vi "close excel file if open.vi"(8 "error in (no error)":errorcluster, 11 "report file path in":path) -> (0 "error out":errorcluster, 3 "report file path out":path)   [LabVIEW 2016]
uses:
  <vilib>/Utility/NIReport.llb/NI_report.lvclass
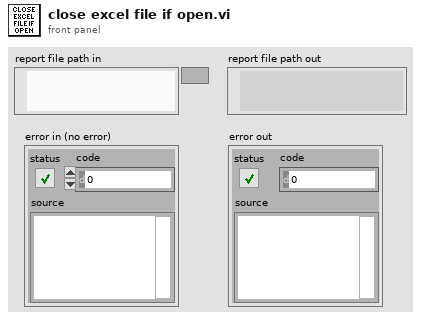
[diagram p1: front panel]
types:
  T1 = enum16{"maximized", "minimized", "normal", "no change"}
  T2 = enum16{"Standard Report", "HTML", "Word", "Excel"}
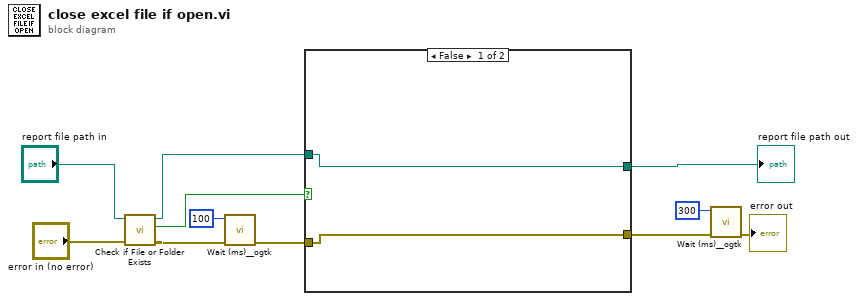
[diagram p0: block diagram]
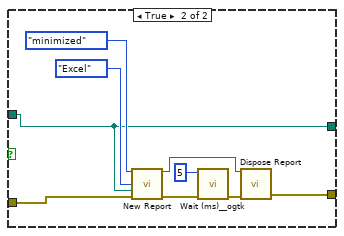
[diagram p2: hidden frame]
diagram:
  n1 = call <vilib>:"Check if File or Folder Exists.vi"("error in (no error)"="error in (no error)", "path"="report file path in") -> ("error out"=w5:errorcluster, "file or folder exists?"=w4:bool, "dup path"=w2:path)  [unwired: 7 in]
  n2 = call "Wait (ms)__ogtk.vi"("error in (no error)"=w5, "milliseconds to wait"=u32 100) -> ("error out"=w7:errorcluster)  [unwired: 8 in, 1 out]
  n3 = case shown="False" w4 {
    tunnel: [w12 w16] -> w11
    tunnel: w7 -> [w12 w15]
    tunnel: w2 -> [w13 w14]
    tunnel: [w13 w14] -> w1
    frame False {
    }
    frame True {
      n4 = call <vilib>:"New Report.vi"("window state (normal)"=T1."minimized", "report type"=T2."Excel", "template (empty)"=w14, "error in (no error)"=w15) -> ("report out"=w18:refnum<class "NI_report.lvclass">, "error out"=w19:errorcluster)  [unwired: 10 in]
      n5 = call "Wait (ms)__ogtk.vi"("error in (no error)"=w19, "milliseconds to wait"=u32 5) -> ("error out"=w22:errorcluster)  [unwired: 8 in, 1 out]
      n6 = call-dynamic "Dispose Report.vi"("report in"=w18, "error in (no error)"=w22) -> ("error out"=w16:errorcluster)  [unwired: 13 in]
    }
  }
  "report file path out" <- w1
  n7 = call "Wait (ms)__ogtk.vi"("error in (no error)"=w11, "milliseconds to wait"=u32 300) -> ("error out"=→"error out":errorcluster)  [unwired: 8 in, 1 out]
